vi "Audio Generate.vi"() -> ()   [LabVIEW 2023]
uses:
  Ctl/QMH Fundamentals - Message Cluster.ctl
  <vilib>/sound2/lvsound2.llb/Sound Data Format.ctl
  <vilib>/sound2/lvsound2.llb/Sampling Mode.ctl
  <vilib>/sound2/lvsound2.llb/Sound Output Write (DBL Single).vi
  <vilib>/sound2/lvsound2.llb/Sound Output Set Volume (Single).vi
panel:
  in  "Quit":bool
  out "生成声音 2":waveform(dbl)(graph)
  in  "频率":dbl=500.0
  in  "Flag":bool
  in  "设备ID":u32
  in  "音量":dbl(slide)=50.0 scale=0.0..100.0
  # "声卡输出测试音"
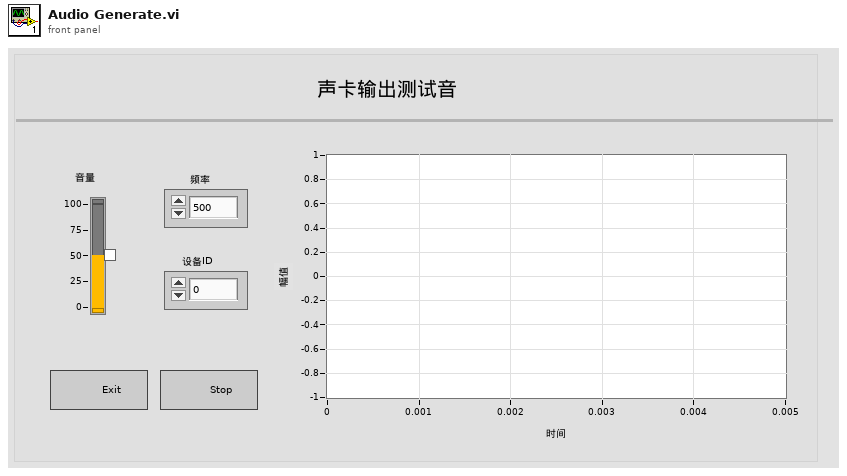
[diagram p1: front panel]
types:
  T1 = typedef "QMH Fundamentals - Message Cluster.ctl" = cluster{"消息":string, "消息数据":variant}
  T2 = typedef "Sound Data Format.ctl" = cluster{"sample rate (S/s)":dbl, "number of channels":i32, "bits per sample":i32}
  T3 = typedef "Sampling Mode.ctl" = i32
  T4 = typedef "Sound Output Task ID.ctl" = u32
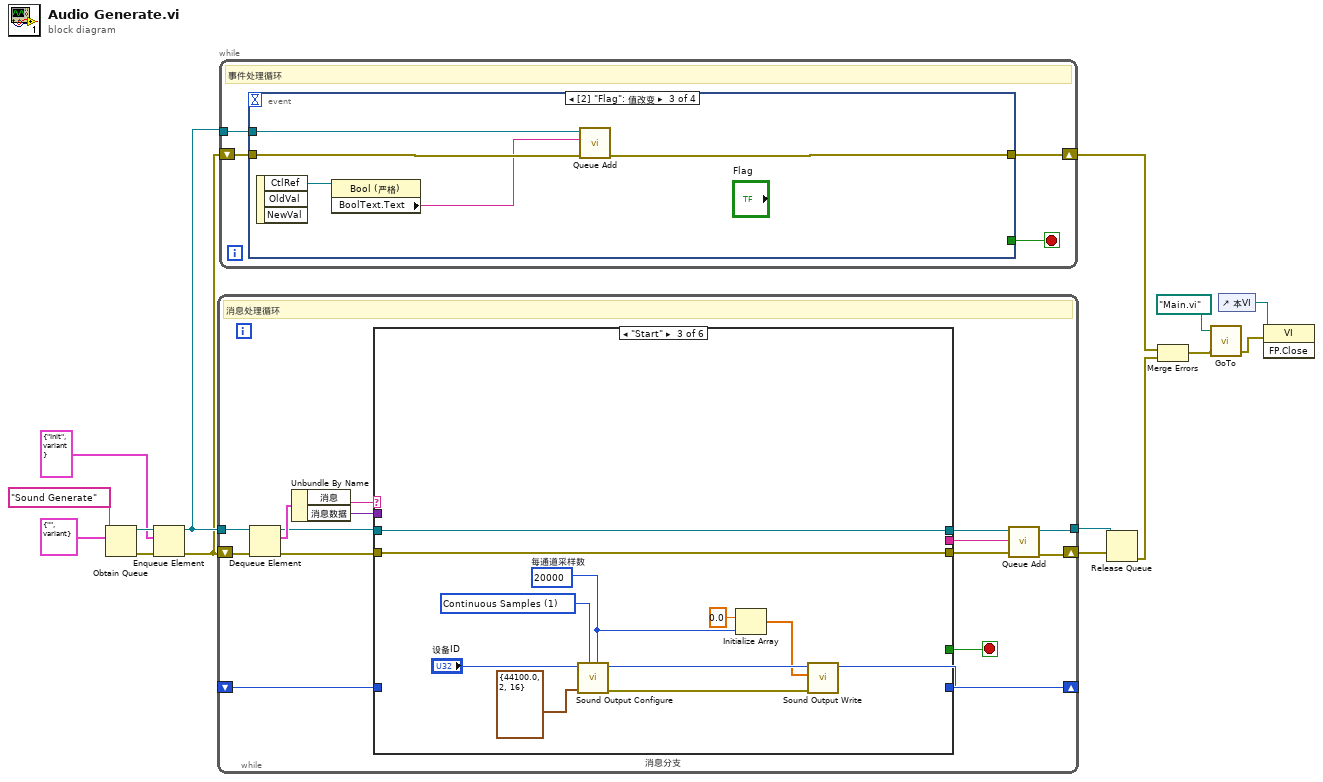
[diagram p0: block diagram]
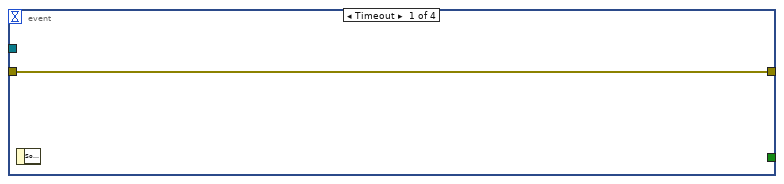
[diagram p2: hidden frame]
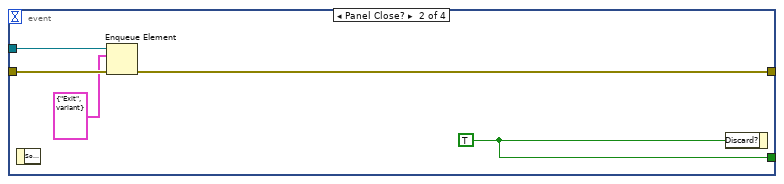
[diagram p3: hidden frame]
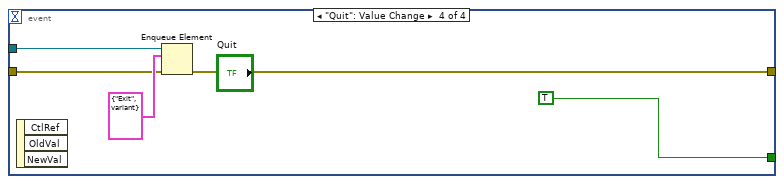
[diagram p4: hidden frame]
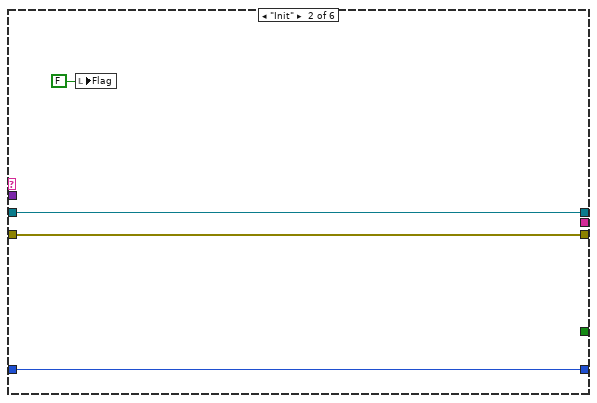
[diagram p6: hidden frame]
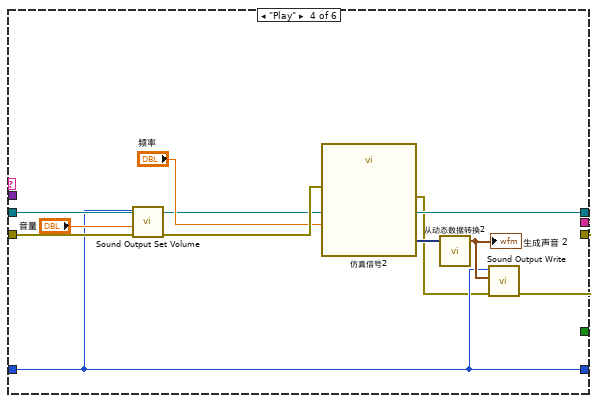
[diagram p7: hidden frame]
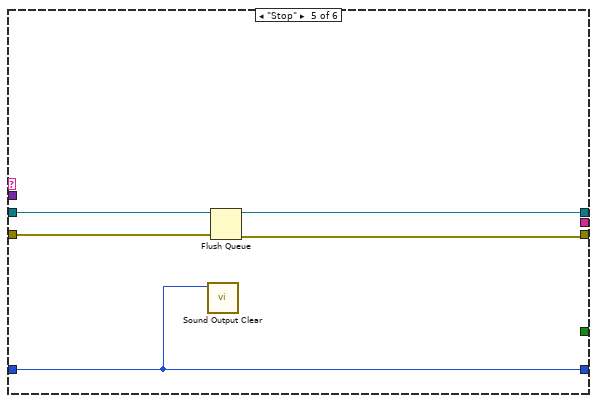
[diagram p8: hidden frame]
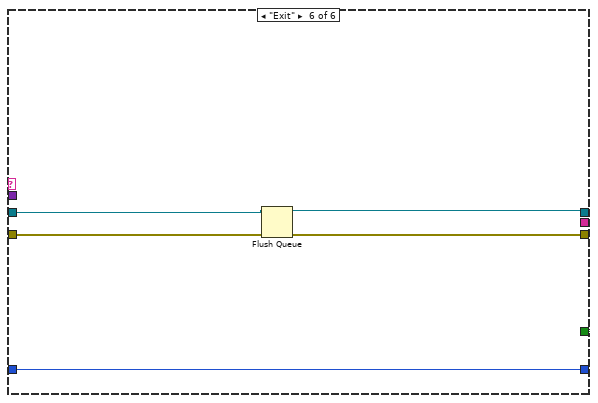
[diagram p9: hidden frame]
diagram:
  n1 = Obtain Queue(name (unnamed)="Sound Generate" ("名称（未命名）"), element data type=T1 {"消息"="", "消息数据"=variant} ("Message Cluster")) -> (queue out=w10:refnum<queue>, error out=w12:errorcluster)  [unwired: 3 in, 1 out]
  n2 = Enqueue Element(queue=w10, element=T1 {"消息"="Init", "消息数据"=variant} ("元素"), error in (no error)=w12) -> (queue out=w8:refnum<queue>, error out=w7:errorcluster)  [unwired: 1 in, 1 out]
  n3 = while {
    tunnel: w8 -> [w29]
    tunnel: [w19] -> w14
    shift-right: [w18] -> w15
    shift-left: w7 -> [w30]
    shift-right: [w23] -> _
    shift-left: _ -> [w22]
    stop <- w17 stop-if-true
    # "消息处理循环"
    n4 = Dequeue Element(queue=w29, error in (no error)=w30) -> (queue out=w27:refnum<queue>, element=w28:T1, error out=w26:errorcluster)  [unwired: 1 in, 1 out]
    n5 = Unbundle By Name(w28) -> ("消息"=w25:string, "消息数据"=w24:variant)
    n6 = case "消息分支" shown="\"Start\"" w25 {
      tunnel: w27 -> [w32 w36 w48 w56 w64 w69]
      tunnel: w26 -> [w33 w37 w49 w60 w63 w70]
      tunnel: [w33 w37 w49 w51 w61 w67] -> w20
      tunnel: [_ _ _ _ _ TRUE] -> w17
      tunnel: w24 -> [_ _ _ _ _ _]
      tunnel: [w32 w36 w48 w56 w62 w68] -> w21
      tunnel: [w31 w35 w39 w53 w65 w66] -> w23
      tunnel: w22 -> [w31 w35 _ w53 w65 w66]
      tunnel: [_ _ "Play" ("消息") "Play" ("消息") _ _] -> w16
      frame "eee", Default {
        # "初始化－执行应用的初始化代码。在本范例中所需的初始化为设置显示消息显示控件的值为空字符串。"
      }
      frame "Init" {
        # "初始化－执行应用的初始化代码。在本范例中所需的初始化为设置显示消息显示控件的值为空字符串。"
        n7 = local write "Flag"(FALSE ("Flag")) -> ()
      }
      frame "Start" {
        w40 = 20000  # 每通道采样数
        w41 = T3 1 items=["Finite Samples", "Continuous Samples"] ("sample mode")
        n8 = call <vilib>:"Sound Output Configure.vi"("number of samples/ch"=w40, "sample mode"=w41, "sound format"=T2 {"sample rate (S/s)"=44100.0, "number of channels"=2, "bits per sample"=16} ("Sound Format"), "device ID"="设备ID") -> ("error out"=w45:errorcluster, "task ID"=w46:T4)  [unwired: 6 in]
        n9 = Initialize Array(0.0 ("element"), w40) -> (w43:dbl[])
        n10 = call-poly <vilib>:"Sound Output Write.vi"("error in (no error)"=w45, "data"=w43, "task ID"=w46) -> ("task ID out"=w39:T4)  [unwired: 7 in, 1 out]
      }
      frame "Play" {
        n11 = call-poly <vilib>:"Sound Output Set Volume.vi"("error in (no error)"=w60, "volume"="音量", "task ID"=w53) -> ("error out"=w58:errorcluster)  [unwired: 7 in, 1 out]
        n12 = call "仿真信号2"("Frequency"="频率", "error in (no error)"=w58) -> ("Sine"=w55:dynamicdata, "error out"=w52:errorcluster)  [unwired: 12 in]
        n13 = call "从动态数据转换2"("Dynamic Data Type"=w55) -> ("Waveform"=w54:waveform(dbl))  [unwired: 3 in]
        "生成声音 2" <- w54
        n14 = call-poly <vilib>:"Sound Output Write.vi"("error in (no error)"=w52, "data"=w54, "task ID"=w53) -> ("error out"=w51:errorcluster)  [unwired: 7 in, 1 out]
      }
      frame "Stop" {
        n15 = call <vilib>:"Sound Output Clear.vi"("task ID"=w65) -> ()  [unwired: 10 in, 1 out]
        n16 = Flush Queue(queue=w64, error in (no error)=w63) -> (queue out=w62:refnum<queue>, error out=w61:errorcluster)  [unwired: 1 out]
      }
      frame "Exit" {
        # "退出－退出应用程序。由于此消息以优先级消息（此消息位于队列的前端）发送，且循环待停止，清理代码应在此处运行。不会处理此队列中的其他消息。"
        n17 = Flush Queue(queue=w69, error in (no error)=w70) -> (queue out=w68:refnum<queue>, error out=w67:errorcluster)  [unwired: 1 out]
      }
    }
    n18 = call "Queue Add.vi"("错误输入（无错误）"=w20, "消息"=w16, "队列输入"=w21) -> ("错误输出"=w18:errorcluster, "队列输出"=w19:refnum<queue>)  [unwired: 7 in]
  }
  n19 = while {
    tunnel: w8 -> [w75]
    shift-right: [w72] -> w5
    shift-left: w7 -> [w73]
    stop <- w74 stop-if-true
    # "事件处理循环"
    n20 = event shown="[2] \"Flag\": 值改变" {
      selector: _ -> [_ _ _ _]
      dyn-events: _ -> [_ _ _ _]
      timeout: _ -> [_ _ _ _]
      tunnel: [_ w81 _ TRUE ("放弃？")] -> w74
      tunnel: w75 -> [_ w80 w83 w90]
      tunnel: [w76 w78 w85 w88] -> w72
      tunnel: w73 -> [w76 w79 w84 w89]
      event Timeout {
        n21 = event-data() -> ()  [unwired: 1 in, 1 out]
      }
      event Panel Close? {
        w81 = TRUE ("放弃？")
        n22 = event-data() -> ()  [unwired: 1 in, 1 out]
        n23 = Enqueue Element(queue=w80, element=T1 {"消息"="Exit", "消息数据"=variant} ("元素"), error in (no error)=w79) -> (error out=w78:errorcluster)  [unwired: 1 in, 2 out]
        n24 = event-data("Discard?"=w81) -> ()  [unwired: 1 in, 1 out]
      }
      event "Flag": Value Change {
        n25 = event-data() -> ("CtlRef"=w86:refnum<vi>)  [unwired: 1 in, 2 out]
        n26 = property class="Bool (严格)"(reference=w86) -> ("BoolText.Text"=w82:string)  [unwired: 1 in, 2 out]
        n27 = call "Queue Add.vi"("错误输入（无错误）"=w84, "消息"=w82, "队列输入"=w83) -> ("错误输出"=w85:errorcluster)  [unwired: 7 in, 1 out]
      }
      event "Quit": Value Change {
        n28 = event-data() -> ()  [unwired: 1 in, 3 out]
        n29 = Enqueue Element(queue=w90, element=T1 {"消息"="Exit", "消息数据"=variant} ("元素"), error in (no error)=w89) -> (error out=w88:errorcluster)  [unwired: 1 in, 2 out]
      }
    }
  }
  n30 = Release Queue(queue=w14, error in (no error)=w15) -> (error out=w4:errorcluster)  [unwired: 1 in, 2 out]
  n31 = Merge Errors(w5, w4) -> (w3:errorcluster)
  n32 = call "GoTo.vi"("错误输入（无错误）"=w3, "名称或相对路径"=path "Main.vi") -> ("错误输出"=w1:errorcluster)  [unwired: 3 in]
  n33 = control-ref of="本VI"() -> (w6:refnum<vi>)
  n34 = invoke class="VI" method="FP.Close"(reference=w6, error in=w1) -> ()  [unwired: 1 in, 3 out]
